vi "ImagetoZ.vi"(9 "queue out":refnum<queue>, 11 "Z":T1) -> (3 "ROI.Z":T1)   [LabVIEW 2016]
uses:
  controls/ModeEnum.ctl
  controls/Microscope Settings.ctl
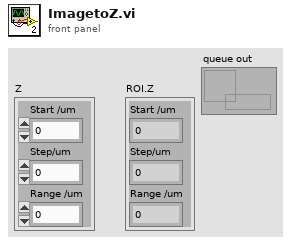
[diagram p1: front panel]
types:
  T1 = cluster{"Start /um":dbl, "Step/um":dbl, "Range /um":dbl}
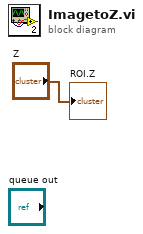
[diagram p0: block diagram]
diagram:
  "ROI.Z" <- "Z"
